vi "Set Cell_wbk_string.vi"(7 "Value":string, 8 "error in (no error)":errorcluster, 9 "Column":i32, 10 "Row":i32, 11 "Sheet":refnum<k24>) -> (0 "error out":errorcluster, 3 "Sheet Out":refnum<k24>)   [LabVIEW 2013]
uses:
  C:/Users/Matt/Downloads/NPOI/LabVIEW/NPOI 2.1.1 dotnet2/NPOI.dll
  Users/Matt/Downloads/NPOI/LabVIEW/NPOI 2.1.1 dotnet2/NPOI.dll
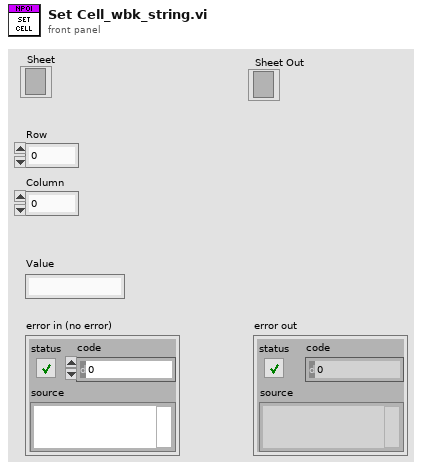
[diagram p1: front panel]
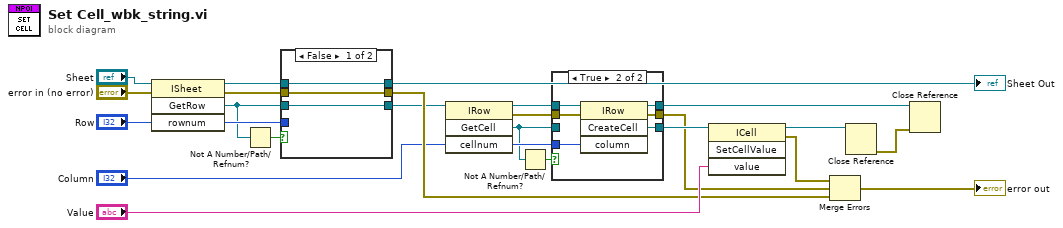
[diagram p0: block diagram]
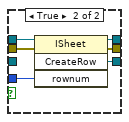
[diagram p3: hidden frame]
diagram:
  n1 = invoke class="ISheet" method="GetRow"(reference="Sheet", error in="error in (no error)", "rownum"="Row") -> (reference out=w14:refnum<k24>, error out=w12:errorcluster, "GetRow"=w10:refnum<k24>)  [unwired: 1 in, 1 out]
  n2 = Not A Number/Path/Refnum?(number/path/refnum=w10) -> (NaN/Path/Refnum?=w16:bool)
  n3 = case shown="False" w16 {
    tunnel: w10 -> [w26 _]
    tunnel: [w26 w32] -> w9
    tunnel: "Row" -> [_ w31]
    tunnel: w14 -> [w25 w30]
    tunnel: [w25 w29] -> w13
    tunnel: w12 -> [w24 w28]
    tunnel: [w24 w27] -> w11
    frame False {
    }
    frame True {
      n4 = invoke class="ISheet" method="CreateRow"(reference=w30, error in=w28, "rownum"=w31) -> (reference out=w29:refnum<k24>, error out=w27:errorcluster, "CreateRow"=w32:refnum<k24>)  [unwired: 1 in, 1 out]
    }
  }
  "Sheet Out" <- w13
  n5 = invoke class="IRow" method="GetCell"(reference=w9, "cellnum"="Column") -> (reference out=w6:refnum<k24>, error out=w4:errorcluster, "GetCell"=w1:refnum<k24>)  [unwired: 2 in, 1 out]
  n6 = Not A Number/Path/Refnum?(number/path/refnum=w1) -> (NaN/Path/Refnum?=w2:bool)
  n7 = case shown="True" w2 {
    tunnel: w1 -> [w34 _]
    tunnel: [w34 w40] -> w7
    tunnel: "Column" -> [_ w39]
    tunnel: w6 -> [w33 w38]
    tunnel: [w33 w37] -> w5
    tunnel: [_ w36] -> w3
    tunnel: w4 -> [_ w35]
    frame False {
    }
    frame True {
      n8 = invoke class="IRow" method="CreateCell"(reference=w38, error in=w35, "column"=w39) -> (reference out=w37:refnum<k24>, error out=w36:errorcluster, "CreateCell"=w40:refnum<k24>)  [unwired: 1 in, 1 out]
    }
  }
  n9 = invoke class="ICell" method="SetCellValue"(reference=w7, "value"="Value") -> (reference out=w21:refnum<k24>, error out=w18:errorcluster)  [unwired: 2 in, 2 out]
  n10 = Merge Errors(w18, w3, w11) -> (→"error out":errorcluster)
  n11 = Close Reference(reference=w21) -> (error out=w17:errorcluster)  [unwired: 1 in]
  n12 = Close Reference(reference=w5, error in (no error)=w17) -> ()  [unwired: 1 out]
